vi "SEA-9811_ReceiverAndTransmitter_FPGA.vi"() -> ()   [LabVIEW 2017]
doc: "This example demonstrates the receiver's functionality. ARINC data can be received with up to 8 channels which can be configured regarding high- or low-speed data rate, label recognition, parity check, decoder functions or label bit order (CONFIG). Up to sixteen 8-bit labels can be stored for label recognition. Duplicate values if you need fewer labels. For more details, look at the RT frontend example.\n\nCopyright (c) 2013-2019 S.E.A. Datentechnik GmbH, Germany"
uses:
  <vilib>/rvi/eio/common/nirviEmuTemplateMethod_errors.vi
  <vilib>/eio/EIOPropertyNode/EIOPropertyNode.xnode
  <vilib>/eio/EIOMethodNode/EIOMethodNode.xnode
  <vilib>/eio/EIONode/EIONode.xnode
  <vilib>/rvi/DataTransferAndStorage/Container/XNode/niFpgaContainer.xnode
  <vilib>/rvi/eio/common/nirviEmuTemplatePropertyGet_errors.vi
  <vilib>/rvi/eio/common/nirviEmuTemplatePropertyGet_noerrors.vi
  <vilib>/rvi/eio/common/nirviEmuTemplatePropertySet_errors.vi
  <vilib>/rvi/eio/common/nirviEmuTemplatePropertySet_noerrors.vi
  <vilib>/rvi/interface/RandomDataEmulation/nirviRandomDataFpgaReadWriteTemplate.vi
panel:
  out "Rx Status":u16 format="%016b"
  out "Tx Status":u8 format="%08b"
  in  "Tx Data":u32=305419896 format="%08x"
  in  "Tx Config Data (TCR)":u16=8192 format="%04x"
  in  "Transmit Data":bool
  out "DMA Overflow":bool
  in  "Rx Label Filter":T1 {"Label 00" format="%02x"; "Label 01" format="%02x"; "Label 02" format="%02x"; "Label 03" format="%02x"; "Label 04" format="%02x"; "Label 05" format="%02x"; "Label 06" format="%02x"; "Label 07" format="%02x"; "Label 08" format="%02x"; "Label 09" format="%02x"; "Label 10" format="%02x"; "Label 11" format="%02x"; "Label 12" format="%02x"; "Label 13" format="%02x"; "Label 14" format="%02x"; "Label 15" format="%02x"}
  in  "Rx Channel Number":u8 max=7 step=1
  in  "Rx Config Data (RCR)":u16=32 format="%04x"
  # "Please refer to VI description for instructions!"
  # "Receiver Configuration"
  # "DMA Status"
  # "Transmitter"
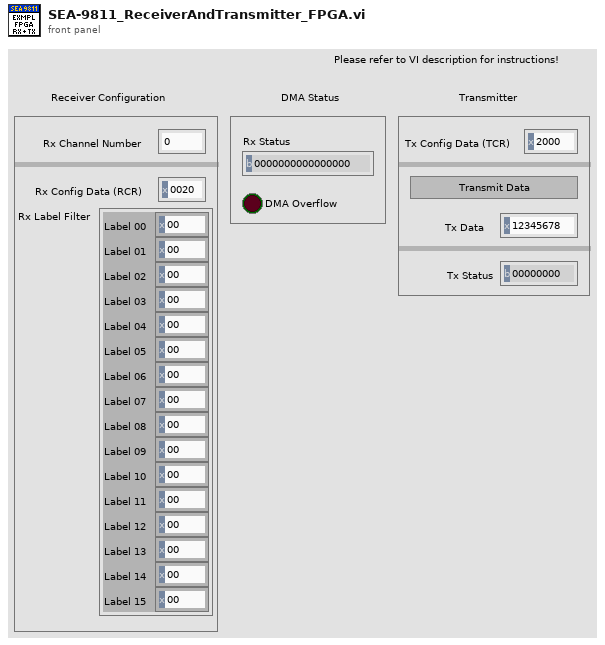
[diagram p1: front panel]
types:
  T1 = cluster{"Label 00":u8, "Label 01":u8, "Label 02":u8, "Label 03":u8, "Label 04":u8, "Label 05":u8, "Label 06":u8, "Label 07":u8, "Label 08":u8, "Label 09":u8, "Label 10":u8, "Label 11":u8, "Label 12":u8, "Label 13":u8, "Label 14":u8, "Label 15":u8}
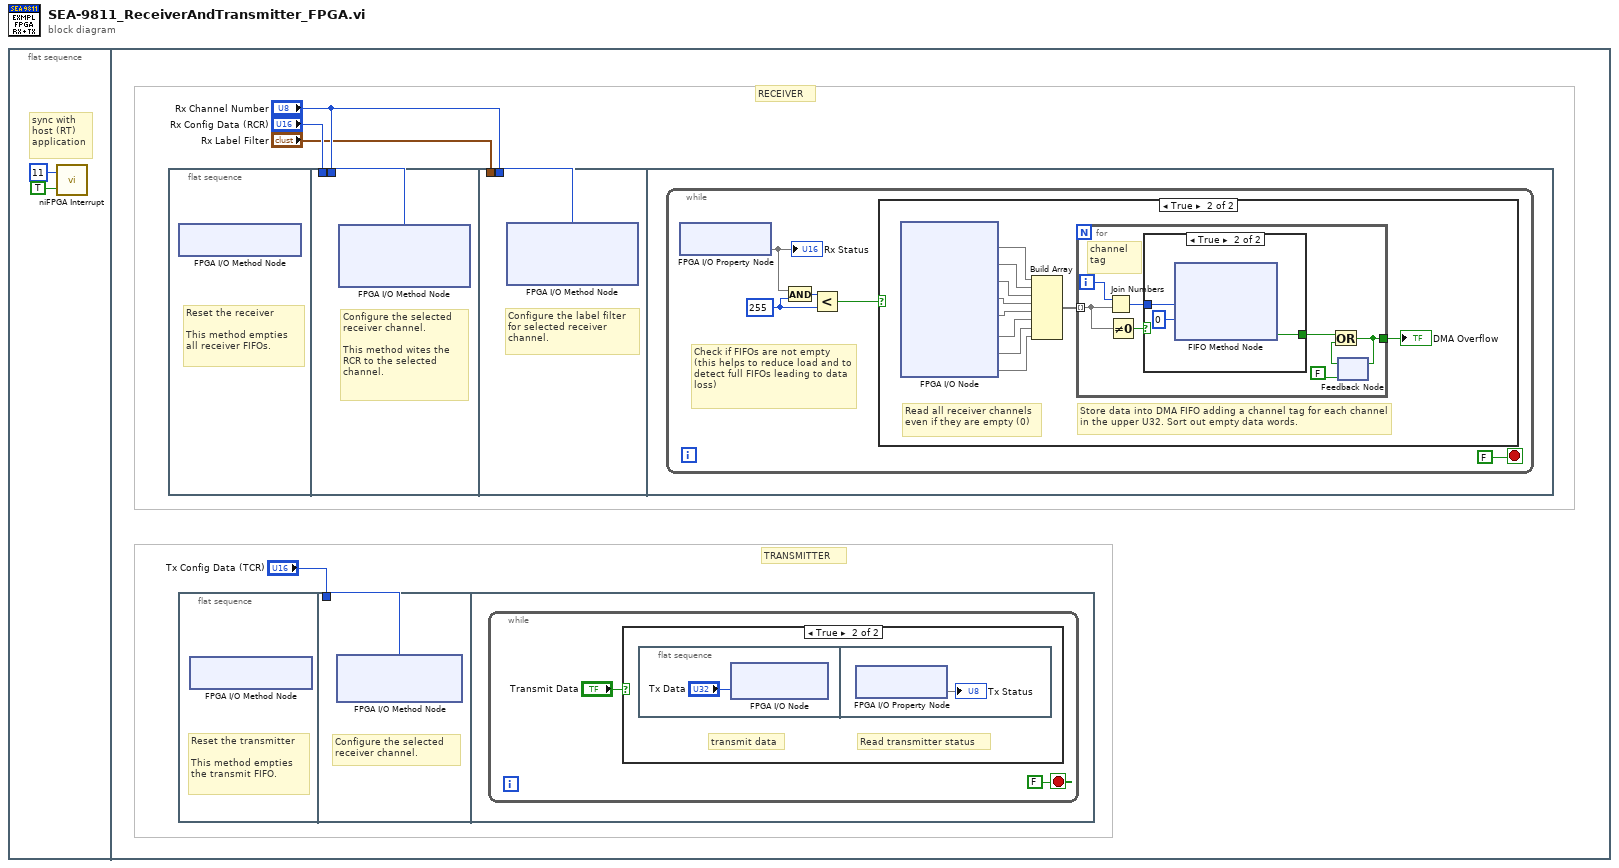
[diagram p0: block diagram]
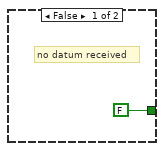
[diagram p4: hidden frame]
diagram:
  n1 = flat-sequence {
    frame #0 {
      # "sync with\nhost (RT)\napplication"
      n2 = call <vilib>:"niFPGA Interrupt.vi"("Wait Until Cleared (F)"=TRUE ("Wait Until Cleared"), "IRQ Number (0)"=u8 11 ("IRQ Number")) -> ()  [unwired: 1 in]
    }
    frame #1 {
      # "TRANSMITTER"
      # "RECEIVER"
      n3 = flat-sequence {
        tunnel: "Rx Channel Number" -> [w13]
        tunnel: "Rx Config Data (RCR)" -> [w12]
        tunnel: "Rx Channel Number" -> [w15]
        tunnel: "Rx Label Filter" -> [w14]
        frame #0 {
          # "Reset the receiver\n\nThis method empties\nall receiver FIFOs."
          n4 = xnode "FPGA I/O Method Node"() -> ()  [unwired: 1 in, 1 out]
        }
        frame #1 {
          # "Configure the selected\nreceiver channel.\n\nThis method wites the\nRCR to the selected\nchannel."
          n5 = xnode "FPGA I/O Method Node"("Channel Number"=w13, "Control Register"=w12) -> ()  [unwired: 1 in, 1 out]
        }
        frame #2 {
          # "Configure the label filter\nfor selected receiver\nchannel."
          n6 = xnode "FPGA I/O Method Node"("Channel Number"=w15, "Label Filter"=w14) -> ()  [unwired: 1 in, 1 out]
        }
        frame #3 {
          n7 = while {
            stop <- FALSE stop-if-true
            w17 = u16 255 ("y")
            # "Check if FIFOs are not empty\n(this helps to reduce load and to detect full FIFOs leading to data loss)"
            n8 = xnode "FPGA I/O Property Node"() -> ("Rx Status"=w19)  [unwired: 1 in, 1 out]
            "Rx Status" <- w19
            n9 = And(x=w19, y=w17) -> (x .and. y?=w18:u16)
            n10 = Less?(x=w18, y=w17) -> (x < y?=w16:bool)
            n11 = case shown="True" w16 {
              frame False {
              }
              frame True {
                # "Store data into DMA FIFO adding a channel tag for each channel in the upper U32. Sort out empty data words."
                # "Read all receiver channels even if they are empty (0)"
                n12 = xnode "FPGA I/O Node"() -> ("Mod1/Rx0"=w22, "Mod1/Rx1"=w23, "Mod1/Rx2"=w24, "Mod1/Rx3"=w25, "Mod1/Rx4"=w26, "Mod1/Rx5"=w27, "Mod1/Rx6"=w28, "Mod1/Rx7"=w29)  [unwired: 8 in, 8 out]
                n13 = Build Array(w22, w23, w24, w25, w26, w27, w28, w29) -> (w21:void[])
                n14 = for {
                  tunnel: w21 -> [w32] mode=indexing
                  tunnel: [w35] -> w30
                  i -> [w31]
                  # "channel\ntag"
                  n15 = Join Numbers(hi=w31, lo=w32) -> ((hi.lo)=w33:u64)
                  n16 = Not Equal To 0?(x=w32) -> (x != 0?=w34:bool)
                  n17 = case shown="True" w34 {
                    tunnel: [FALSE ("Timed Out?") w41] -> w36
                    tunnel: w33 -> [_ w40]
                    frame False {
                      # "no datum received"
                    }
                    frame True {
                      n18 = xnode ("FIFO Method Node")("Element"=w40, "Timeout"=0) -> ("Timed Out?"=w41:bool)  [unwired: 1 in, 1 out]
                    }
                  }
                  n19 = feedback #1(FALSE) -> (w37:bool)
                  n20 = Or(x=w36, y=w37) -> (x .or. y?=w35:bool)
                  n21 = feedback-in #1(w35) -> ()
                }
                "DMA Overflow" <- w30
              }
            }
          }
        }
      }
      n22 = flat-sequence {
        tunnel: "Tx Config Data (TCR)" -> [w7]
        frame #0 {
          # "Reset the transmitter\n\nThis method empties\nthe transmit FIFO."
          n23 = xnode "FPGA I/O Method Node"() -> ()  [unwired: 1 in, 1 out]
        }
        frame #1 {
          # "Configure the selected\nreceiver channel."
          n24 = xnode "FPGA I/O Method Node"("Control Register"=w7) -> ()  [unwired: 1 in, 1 out]
        }
        frame #2 {
          n25 = while {
            stop <- FALSE stop-if-true
            n26 = case shown="True" "Transmit Data" {
              frame False {
              }
              frame True {
                # "Read transmitter status"
                # "transmit data"
                n27 = flat-sequence {
                  frame #0 {
                    n28 = xnode "FPGA I/O Node"("Mod1/Tx0"="Tx Data") -> ()  [unwired: 1 in, 1 out]
                  }
                  frame #1 {
                    n29 = xnode "FPGA I/O Property Node"() -> ("Tx Status"=→"Tx Status")  [unwired: 1 in, 1 out]
                  }
                }
              }
            }
          }
        }
      }
    }
  }
